vi "SetDir.vi"(0 "reference in":refnum<class "ConfigJSON.lvclass">, 5 "Config Dir":path) -> (4 "JSON":refnum<class "ConfigJSON.lvclass">)   [LabVIEW 2019, in "ConfigJSON.lvclass"]
uses:
  ConfigJSON.lvclass
  ConfigJSON.lvclass/ConfigJSON.ctl
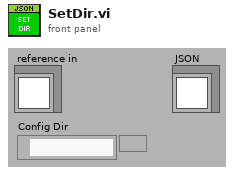
[diagram p1: front panel]
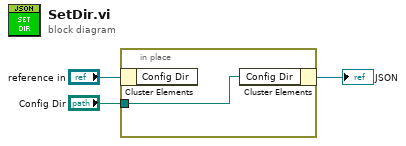
[diagram p0: block diagram]
diagram:
  n1 = in-place {
    in-place-border: "Config Dir" -> [w4]
    n2 = in-place-cluster #1("reference in") -> ()  [unwired: 1 out]
    n3 = in-place-cluster #1("Config Dir"=w4) -> (→"JSON":refnum<class "ConfigJSON.lvclass">)
  }
